vi "Create Subscriber.vi"(8 "error in (no error)":errorcluster, 9 "Default Value":dbl, 10 "Name":string, 11 "RTFIFODouble in":refnum<class "RTFIFODouble.lvclass">) -> (0 "error out":errorcluster, 3 "RTFIFODouble out":refnum<class "RTFIFODouble.lvclass">)   [LabVIEW 2021, in "RTFIFODouble.lvclass"]
uses:
  RTFIFODouble.lvclass
  D:/dev/CIF-LVCore/src/Channels/CIFChannels/CIFChannels.lvclass
  CIFChannels/Typedef/Direction.ctl
  CIFChannels/Typedef/Disconnect Behavior.ctl
  CIFChannels/CIFChannels.lvclass/CIFChannels.ctl
  RTFIFODouble.lvclass/RTFIFODouble.ctl
  CIFChannels/Accessors/Write Channel Class.vi
  CIFChannels/Accessors/Write Channel State.vi
  CIFChannels/Accessors/Write Direction.vi
  CIFChannels/Accessors/Write Disconnect Behavior.vi
  CIFChannels/Accessors/Write Name.vi
  CIFChannels/Accessors/Write Custom Config Data.vi
  <vilib>/Utility/LVClass/Get LV Class Name.vi
  CIFChannels/CIFChannels.lvclass
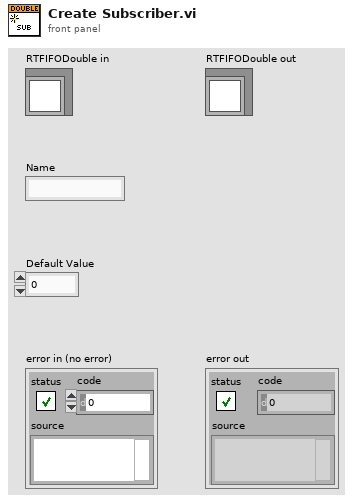
[diagram p1: front panel]
types:
  T1 = typedef "CIFChannels.lvclass/Disconnect Behavior.ctl" = enum16{"Default value", "Last value", "Error with default"}
  T2 = typedef "CIFChannels.lvclass/Direction.ctl" = enum16{"Publisher", "Subscriber"}
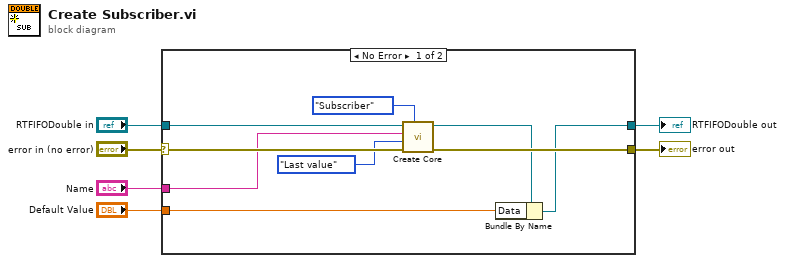
[diagram p0: block diagram]
diagram:
  n1 = case shown="No Error" "error in (no error)" {
    selector: "error in (no error)" -> [w13 w17]
    tunnel: [w10 w17] -> w5
    tunnel: [w7 w16] -> w3
    tunnel: "RTFIFODouble in" -> [w15 w16]
    tunnel: "Name" -> [w11 _]
    tunnel: "Default Value" -> [w8 _]
    frame No Error {
      n2 = call "Create Core.vi"("Direction"=Direction."Subscriber", "error in (no error)"=w13, "Disconnect Behavior"=Disconnect_Behavior."Last value", "Name"=w11, "CIFChannels in"=w15) -> ("error out"=w10:errorcluster, "CIFChannels out"=w9:refnum<class "RTFIFODouble.lvclass">)  [unwired: 5 in]
      n3 = Bundle By Name(cluster=w9, "Data"=w8) -> (w7:refnum<class "RTFIFODouble.lvclass">)
    }
    frame Error {
    }
  }
  "error out" <- w5
  "RTFIFODouble out" <- w3
